vi "Read PlatMods.vi"(8 "error in (no error)":errorcluster, 11 "ControlDragOverMsg In":refnum<class "ControlDragOverMsg.lvclass">) -> (0 "error out":errorcluster, 2 "PlatMods":T1, 3 "ControlDragOverMsg Out":refnum<class "ControlDragOverMsg.lvclass">)   [LabVIEW 2020, in "MVA Framework.lvlib" / "ActorEvents.lvlib" / "ControlDragOverMsg.lvclass"]
uses:
  ControlDragOverMsg.lvclass
  ControlDragOverMsg.lvclass/ControlDragOverMsg.ctl
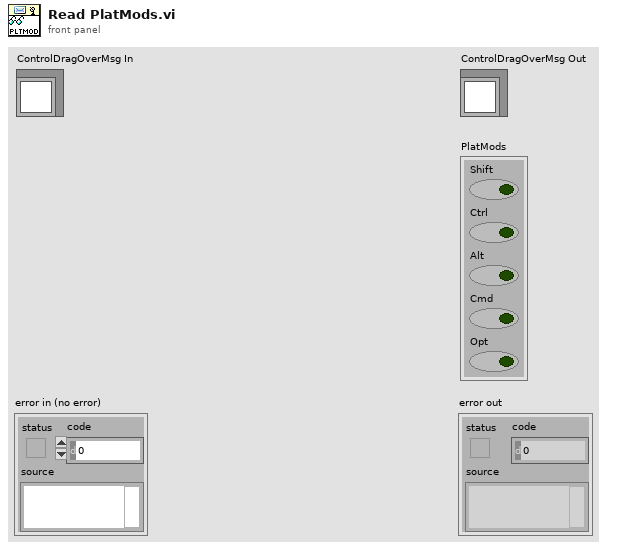
[diagram p1: front panel]
types:
  T1 = cluster{"Shift":bool, "Ctrl":bool, "Alt":bool, "Cmd":bool, "Opt":bool}
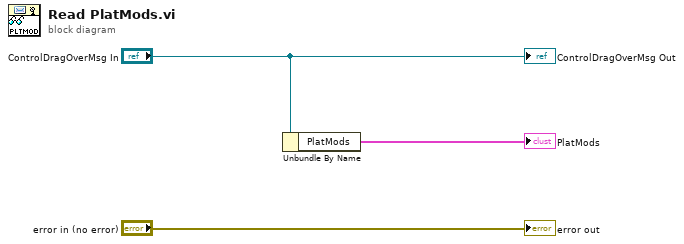
[diagram p0: block diagram]
diagram:
  n1 = Unbundle By Name("ControlDragOverMsg In") -> ("PlatMods"=→"PlatMods":T1)
  "error out" <- "error in (no error)"
  "ControlDragOverMsg Out" <- "ControlDragOverMsg In"
